vi "Write MODBUS Serial Parameters.vi"(8 "error in (no error)":errorcluster, 10 "MODBUS Serial Parameters":T1={"Mode"=enum."RTU", "Default Slave Address"=111, "MODBUS timeout"=1000, "Baud Rate"=38400, "Parity"=0, "Flow Control"=0} {"Flow Control" items=["None", "XON/XOFF", "RTS/CTS", "XON/XOFF & RTS/CTS", "DTR/DSR", "XON/XOFF & DTR/DSR"]; "Parity" items=["None", "Odd", "Even", "Mark", "Space"]}, 11 "MODBUS in":refnum<class "MODBUS.lvclass">) -> (0 "error out":errorcluster, 3 "MODBUS out":refnum<class "MODBUS.lvclass">)   [LabVIEW 2016, in "MODBUS.lvclass"]
uses:
  MODBUS.lvclass
  MODBUS parameters type.ctl
  MODBUS.lvclass/MODBUS.ctl
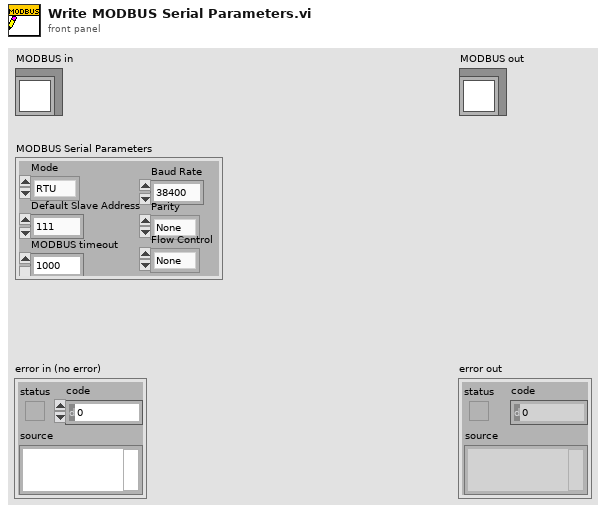
[diagram p1: front panel]
types:
  T1 = typedef "MODBUS parameters type.ctl" = cluster{"Mode":enum16{"RTU", "ASCII"}, "Default Slave Address":u8, "MODBUS timeout":u32, "Baud Rate":u32, "Parity":u16, "Flow Control":u16}
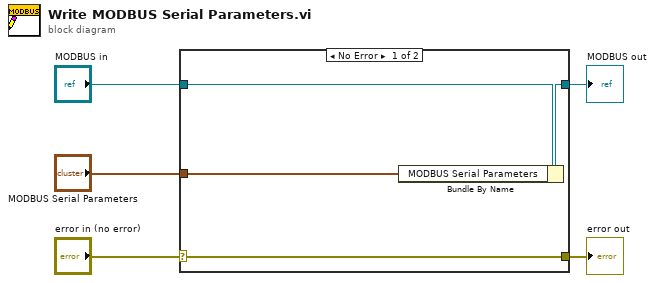
[diagram p0: block diagram]
diagram:
  n1 = case shown="No Error" "error in (no error)" {
    selector: "error in (no error)" -> [w9 w10]
    tunnel: [w9 w10] -> w4
    tunnel: [w7 w11] -> w2
    tunnel: "MODBUS in" -> [w8 w11]
    tunnel: "MODBUS Serial Parameters" -> [w6 _]
    frame No Error {
      n2 = Bundle By Name(cluster=w8, "MODBUS Serial Parameters"=w6) -> (w7:refnum<class "MODBUS.lvclass">)
    }
    frame Error {
    }
  }
  "error out" <- w4
  "MODBUS out" <- w2
